vi "Leap_Detection.vi"(0 "Leap Handle in":T1, 5 "Max distance in":sgl[](array[numeric]), 7 "Not Tracked?":bool, 9 "Calibrate?":bool, 11 "error in (no error)":errorcluster) -> (4 "Leap Handle out":T1, 6 "Max Distance out":dbl[](array[numeric]), 10 "Finger Positions":dbl[](array[numeric]), 15 "error out":errorcluster)   [LabVIEW 2015]
uses:
  <vilib>/MakerHub/Leap/Private/Type Defs/Leap Handle.ctl
  C:/Program Files (x86)/National Instruments/LabVIEW 2015/vi.lib/MakerHub/Leap/Private/Libs/LeapCSharp.NET3.5.dll
  Program Files (x86)/National Instruments/LabVIEW 2015/vi.lib/MakerHub/Leap/Private/Libs/LeapCSharp.NET3.5.dll
  <vilib>/MakerHub/Leap/LMH-Leap.lvlib
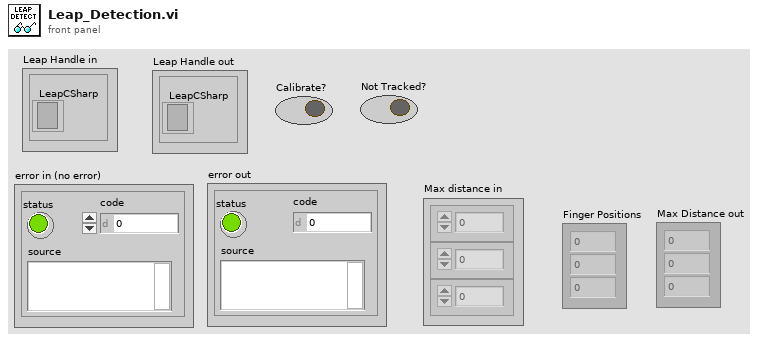
[diagram p1: front panel]
types:
  T1 = typedef "LMH-Leap.lvlib/Leap Handle.ctl" = cluster{"LeapCSharp":refnum<k24>}
  T2 = cluster{"ID":dbl, "X":dbl, "Y":dbl, "Z":dbl, "Length":dbl}[]
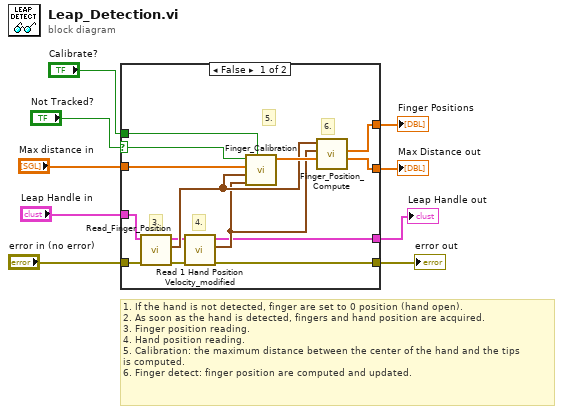
[diagram p0: block diagram]
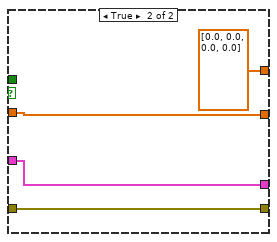
[diagram p2: hidden frame]
diagram:
  # "1. If the hand is not detected, finger are set to 0 position (hand open).\n2. As soon as the hand is detected, fingers and hand position are acquired.\n3. Finger position reading.\n4. Hand position reading.\n5. Calibration: the maximum distance between the center of the hand and the tips\nis computed.\n6. Finger detect: finger position are computed and updated."
  n1 = case shown="False" "Not Tracked?" {
    selector: "Not Tracked?" -> [w13 _]
    tunnel: [w23 dbl[] [0.0, 0.0, 0.0, 0.0] ("Finger position")] -> w9
    tunnel: "Leap Handle in" -> [w22 w25]
    tunnel: "error in (no error)" -> [w21 w24]
    tunnel: [w19 w27] -> w6
    tunnel: "Max distance in" -> [w17 w27]
    tunnel: "Calibrate?" -> [w10 _]
    tunnel: [w12 w24] -> w2
    tunnel: [w11 w25] -> w1
    frame False {
      # "6."
      # "5."
      # "4."
      # "3."
      n2 = call "Read_Finger_Position.vi"("Error In"=w21, "Leap Handle"=w22) -> ("Error Out"=w15:errorcluster, "Finger Positions"=w18:T2, "Leap Handle 2"=w16:T1)  [unwired: 7 in]
      n3 = call "Read 1 Hand Position Velocity_modified.vi"("Error In"=w15, "Leap Handle"=w16) -> ("Error Out"=w12:errorcluster, "Hand Position"=w14:cluster{"X":sgl, "Y":sgl, "Z":sgl}, "Leap Handle"=w11:T1)  [unwired: 6 in, 1 out]
      n4 = call "Finger_Calibration.vi"("Calibrate?"=w10, "Hand Position"=w14, "Finger Positions"=w18, "Max distance in"=w17, "Not Tracked?"=w13) -> ("Max distance out"=w20:dbl[])  [unwired: 6 in]
      n5 = call "Finger_Position_Compute.vi"("Max Distance"=w20, "Hand Position"=w14, "Finger Positions"=w18) -> ("Max Distance out"=w19:dbl[], "Finger position"=w23:dbl[])  [unwired: 7 in]
    }
    frame True {
      # "1."
    }
  }
  "Finger Positions" <- w9
  "Max Distance out" <- w6
  "Leap Handle out" <- w1
  "error out" <- w2
